vi "worker2.vi"(10 "user.xls path":path, 11 "Python version":string) -> (0 "error out":errorcluster, 8 "error In":errorcluster)   [LabVIEW 2020]
uses:
  status/stop software.vi
  status/skip_status.vi
  status/pause2.vi
  status/emergency stop.vi
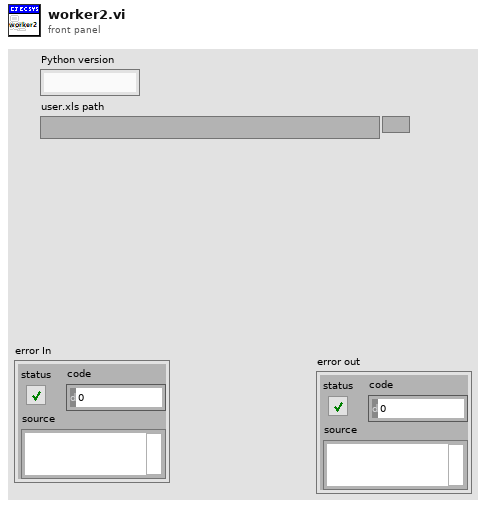
[diagram p1: front panel]
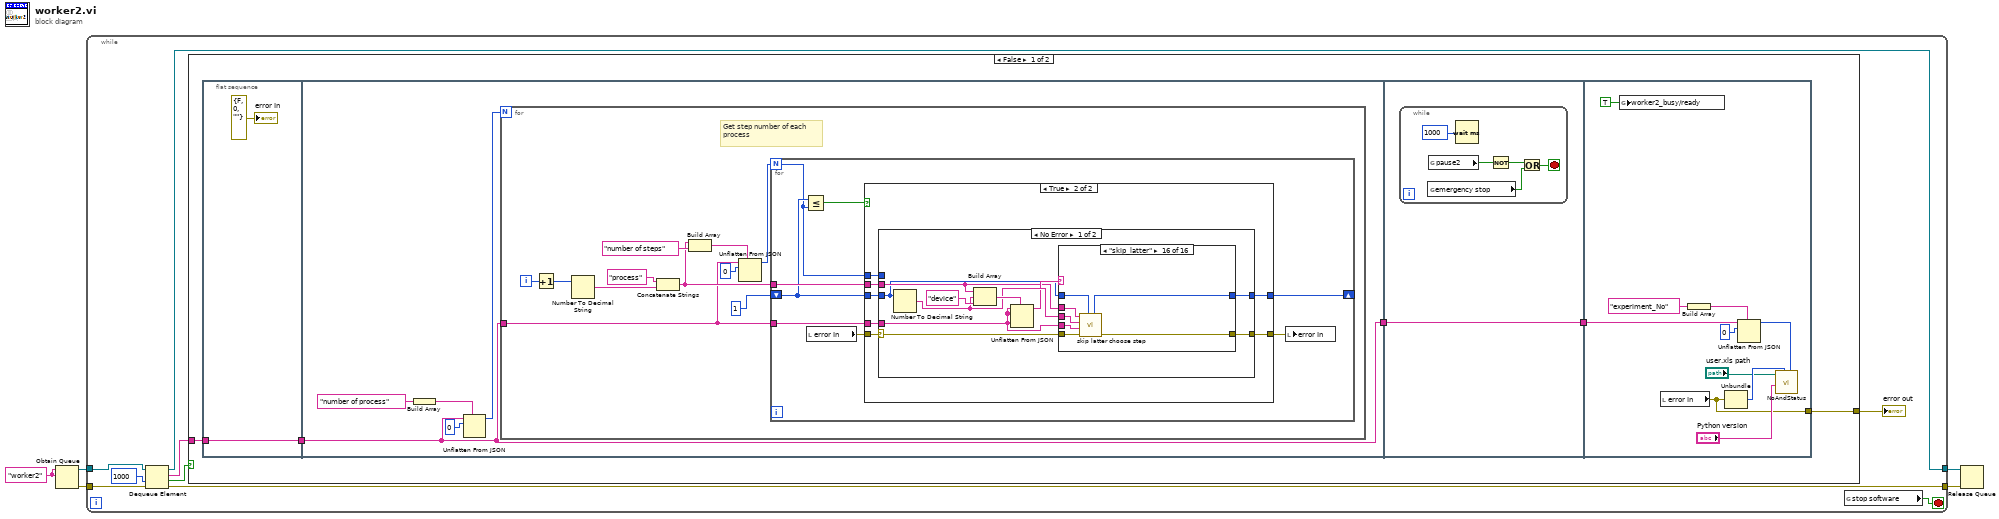
[diagram p0: block diagram]
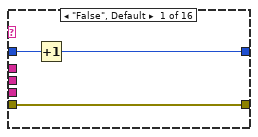
[diagram p3: hidden frame]
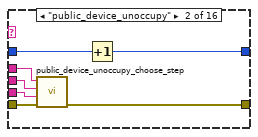
[diagram p4: hidden frame]
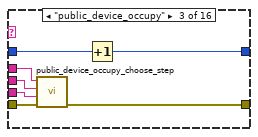
[diagram p5: hidden frame]
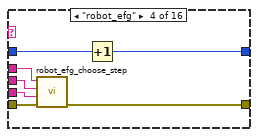
[diagram p6: hidden frame]
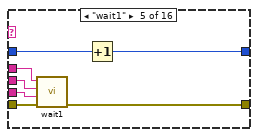
[diagram p7: hidden frame]
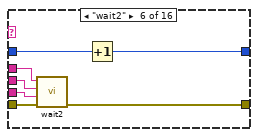
[diagram p8: hidden frame]
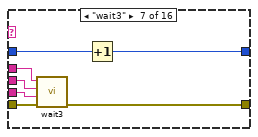
[diagram p9: hidden frame]
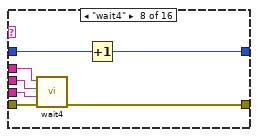
[diagram p10: hidden frame]
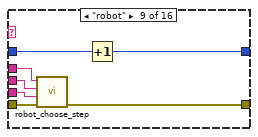
[diagram p11: hidden frame]
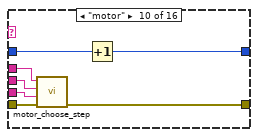
[diagram p12: hidden frame]
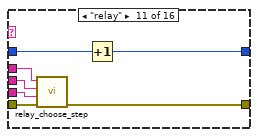
[diagram p13: hidden frame]
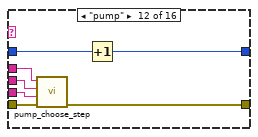
[diagram p14: hidden frame]
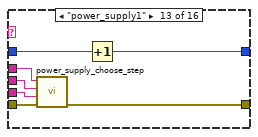
[diagram p15: hidden frame]
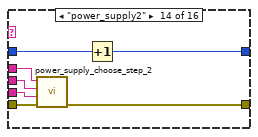
[diagram p16: hidden frame]
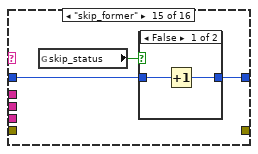
[diagram p17: hidden frame]
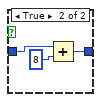
[diagram p18: hidden frame]
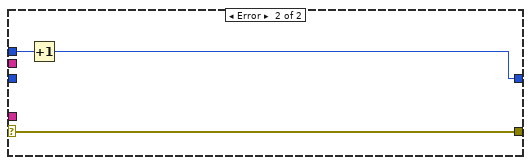
[diagram p19: hidden frame]
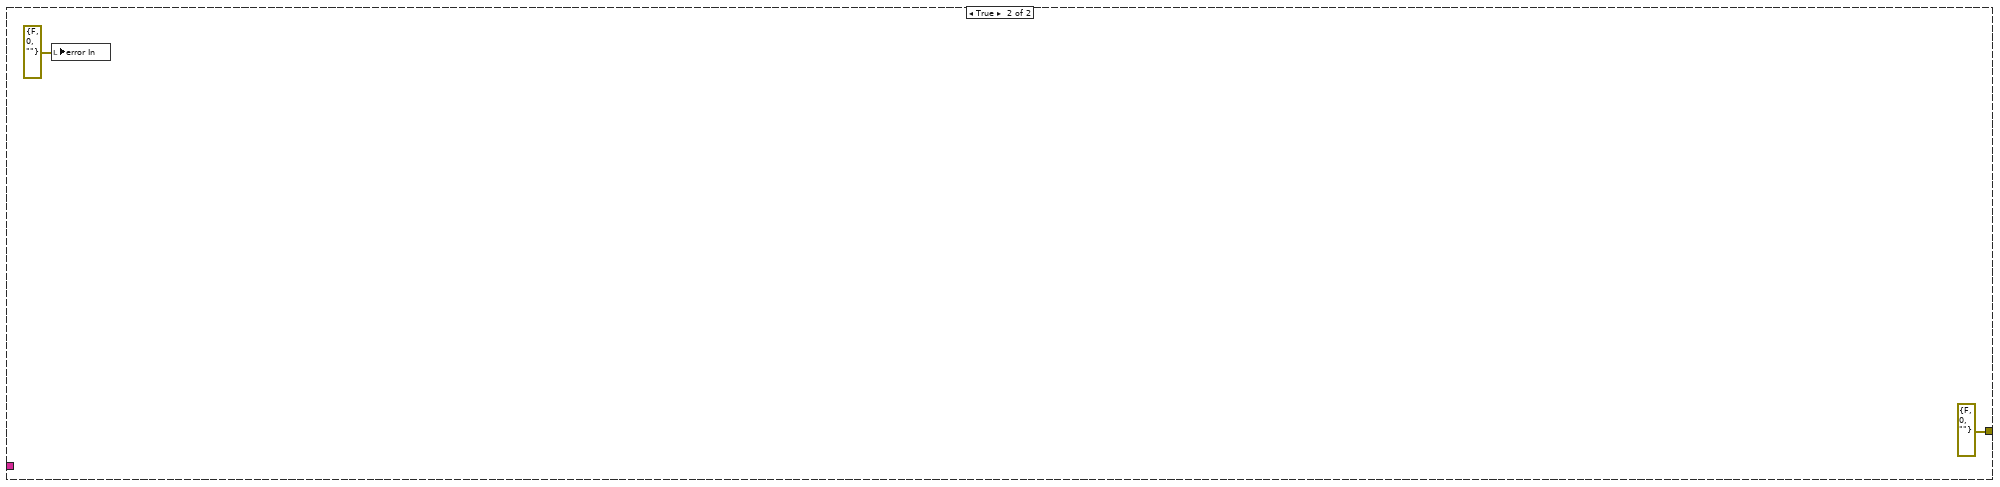
[diagram p20: hidden frame]
diagram:
  w3 = "worker2" ("name (unnamed)")
  n1 = Obtain Queue(name (unnamed)=w3, element data type=w3) -> (queue out=w2:refnum<queue>, error out=w1:errorcluster)  [unwired: 3 in, 1 out]
  n2 = while {
    tunnel: [w11] -> w5
    tunnel: [w10] -> w4
    tunnel: w2 -> [w7]
    tunnel: w1 -> [w6]
    stop <- w9 stop-if-true
    n3 = Dequeue Element(queue=w7, timeout in ms (-1)=1000, error in (no error)=w6) -> (queue out=w11:refnum<queue>, element=w12:string, timed out?=w14:bool, error out=w10:errorcluster)
    n4 = case shown="False" w14 {
      tunnel: w12 -> [w18 _]
      tunnel: [w15 errorcluster {"status"=FALSE, "code"=0, "source"=""} ("error In")] -> w8
      frame False {
        n5 = flat-sequence {
          tunnel: [w21] -> w19
          tunnel: w18 -> [w21]
          tunnel: w19 -> [w22]
          tunnel: [w22] -> w16
          tunnel: [w177] -> w17
          tunnel: w16 -> [w177]
          tunnel: w17 -> [w185]
          tunnel: [w183] -> w15
          frame #0 {
            "error In" <- errorcluster {"status"=FALSE, "code"=0, "source"=""} ("error In")
          }
          frame #1 {
            n6 = Build Array("number of process") -> (w24:string[])
            n7 = Unflatten From JSON(path=w24, JSON string=w22, type and defaults=0) -> (value=w23:i32)  [unwired: 4 in, 1 out]
            n8 = for {
              N: w23 -> [_]
              tunnel: w22 -> [w28]
              i -> [w35]
              # "Get step number of each process"
              n9 = Increment(x=w35) -> (x+1=w30:i32)
              n10 = Number To Decimal String(number=w30) -> (decimal integer string=w33:string)  [unwired: 1 in]
              n11 = Concatenate Strings("process" ("string"), w33) -> (w29:string)
              n12 = Build Array(w29, "number of steps" ("element")) -> (w31:string[])
              n13 = Unflatten From JSON(path=w31, JSON string=w28, type and defaults=0) -> (value=w36:i32)  [unwired: 4 in, 1 out]
              n14 = for {
                N: w36 -> [w38]
                tunnel: w29 -> [w43]
                tunnel: w28 -> [w42]
                shift-right: [w40] -> _
                shift-left: 1 ("Numeric") -> [w39]
                n15 = Less Or Equal?(x=w39, y=w38) -> (x <= y?=w41:bool)
                n16 = local read "error In"() -> (w45:errorcluster)
                n17 = case shown="True" w41 {
                  tunnel: [w47 w54] -> w44
                  tunnel: w45 -> [w47 w53]
                  tunnel: w42 -> [_ w52]
                  tunnel: w39 -> [w46 w51]
                  tunnel: [w46 w50] -> w40
                  tunnel: w38 -> [_ w49]
                  tunnel: w43 -> [_ w48]
                  frame False {
                  }
                  frame True {
                    n18 = case shown="No Error" w53 {
                      selector: w53 -> [w59 w176]
                      tunnel: [w63 w176] -> w54
                      tunnel: w48 -> [w58 _]
                      tunnel: w52 -> [w57 _]
                      tunnel: w51 -> [w55 _]
                      tunnel: [w56 w175] -> w50
                      tunnel: w49 -> [_ w174]
                      frame No Error {
                        n19 = Number To Decimal String(number=w55) -> (decimal integer string=w61:string)  [unwired: 1 in]
                        n20 = Build Array(w58, w61, "device" ("element")) -> (w62:string[])
                        n21 = Unflatten From JSON(path=w62, JSON string=w57, type and defaults=w57) -> (value=w60:string)  [unwired: 4 in, 1 out]
                        n22 = case shown="\"skip_latter\"" w60 {
                          tunnel: w57 -> [_ w71 w78 w88 w92 w99 w107 w114 w120 w127 w134 w144 w149 w155 _ w172]
                          tunnel: [w67 w74 w81 w87 w95 w102 w106 w113 w123 w130 w137 w143 w151 w158 _ w168] -> w63
                          tunnel: w61 -> [_ w72 w79 w85 w93 w100 w108 w115 w121 w128 w135 w141 w148 w156 _ w171]
                          tunnel: w58 -> [_ w73 w80 w86 w94 w101 w109 w116 w122 w129 w136 w142 w150 w157 _ w173]
                          tunnel: w59 -> [w67 w70 w77 w84 w91 w98 w105 w112 w119 w126 w133 w140 w147 w154 _ w167]
                          tunnel: [w66 w69 w76 w82 w90 w97 w104 w111 w118 w125 w132 w139 w146 w153 w159 w169] -> w56
                          tunnel: w55 -> [w65 w68 w75 w83 w89 w96 w103 w110 w117 w124 w131 w138 w145 w152 w160 w170]
                          frame "False", Default {
                            n23 = Increment(x=w65) -> (x+1=w66:i32)
                          }
                          frame "public_device_unoccupy" {
                            n24 = call "public_device_unoccupy_choose_step.vi"("error In"=w70, "JSON string"=w71, "Step order"=w72, "process_ID"=w73) -> ("error IO"=w74:errorcluster)  [unwired: 7 in]
                            n25 = Increment(x=w68) -> (x+1=w69:i32)
                          }
                          frame "public_device_occupy" {
                            n26 = call "public_device_occupy_choose_step.vi"("error In"=w77, "JSON string"=w78, "Step order"=w79, "process_ID"=w80) -> ("error IO"=w81:errorcluster)  [unwired: 7 in]
                            n27 = Increment(x=w75) -> (x+1=w76:i32)
                          }
                          frame "robot_efg" {
                            n28 = call "robot_efg_choose_step.vi"("error In"=w84, "JSON string"=w88, "Step order"=w85, "process_ID"=w86) -> ("error IO"=w87:errorcluster)  [unwired: 7 in]
                            n29 = Increment(x=w83) -> (x+1=w82:i32)
                          }
                          frame "wait1" {
                            n30 = call "wait1.vi"("error In"=w91, "JSON string"=w92, "Step order"=w93, "process_ID"=w94) -> ("error IO"=w95:errorcluster)  [unwired: 7 in]
                            n31 = Increment(x=w89) -> (x+1=w90:i32)
                          }
                          frame "wait2" {
                            n32 = call "wait2.vi"("error In"=w98, "JSON string"=w99, "Step order"=w100, "process_ID"=w101) -> ("error IO"=w102:errorcluster)  [unwired: 7 in]
                            n33 = Increment(x=w96) -> (x+1=w97:i32)
                          }
                          frame "wait3" {
                            n34 = call "wait3.vi"("error In"=w105, "JSON string"=w107, "Step order"=w108, "process_ID"=w109) -> ("error IO"=w106:errorcluster)  [unwired: 7 in]
                            n35 = Increment(x=w103) -> (x+1=w104:i32)
                          }
                          frame "wait4" {
                            n36 = call "wait4.vi"("error In"=w112, "JSON string"=w114, "Step order"=w115, "process_ID"=w116) -> ("error IO"=w113:errorcluster)  [unwired: 7 in]
                            n37 = Increment(x=w110) -> (x+1=w111:i32)
                          }
                          frame "robot" {
                            n38 = call "robot_choose_step.vi"("error In"=w119, "JSON string"=w120, "Step order"=w121, "process_ID"=w122) -> ("error IO"=w123:errorcluster)  [unwired: 7 in]
                            n39 = Increment(x=w117) -> (x+1=w118:i32)
                          }
                          frame "motor" {
                            n40 = call "motor_choose_step.vi"("error In"=w126, "JSON string"=w127, "Step order"=w128, "process_ID"=w129) -> ("error IO"=w130:errorcluster)  [unwired: 7 in]
                            n41 = Increment(x=w124) -> (x+1=w125:i32)
                          }
                          frame "relay" {
                            n42 = call "relay_choose_step.vi"("error In"=w133, "JSON string"=w134, "Step order"=w135, "process_ID"=w136) -> ("error IO"=w137:errorcluster)  [unwired: 7 in]
                            n43 = Increment(x=w131) -> (x+1=w132:i32)
                          }
                          frame "pump" {
                            n44 = call "pump_choose_step.vi"("error In"=w140, "JSON string"=w144, "Step order"=w141, "process_ID"=w142) -> ("error IO"=w143:errorcluster)  [unwired: 7 in]
                            n45 = Increment(x=w138) -> (x+1=w139:i32)
                          }
                          frame "power_supply1" {
                            n46 = call "power_supply_choose_step.vi"("error In"=w147, "JSON string"=w149, "Step order"=w148, "process_ID"=w150) -> ("error IO"=w151:errorcluster)  [unwired: 7 in]
                            n47 = Increment(x=w145) -> (x+1=w146:i32)
                          }
                          frame "power_supply2" {
                            n48 = call "power_supply_choose_step_2.vi"("error In"=w154, "JSON string"=w155, "Step order"=w156, "process_ID"=w157) -> ("error IO"=w158:errorcluster)  [unwired: 7 in]
                            n49 = Increment(x=w152) -> (x+1=w153:i32)
                          }
                          frame "skip_former" {
                            n50 = global read "skip_status.vi" "skip_status"() -> (w161:bool)
                            n51 = case shown="False" w161 {
                              tunnel: w160 -> [w162 w166]
                              tunnel: [w163 w164] -> w159
                              frame False {
                                n52 = Increment(x=w162) -> (x+1=w163:i32)
                              }
                              frame True {
                                n53 = Add(x=w166, y=8) -> (x+y=w164:i32)
                              }
                            }
                          }
                          frame "skip_latter" {
                            n54 = call "skip latter choose step.vi"("step number"=w170, "error In"=w167, "JSON string"=w172, "Step order"=w171, "process_ID"=w173) -> ("error IO"=w168:errorcluster, "step number after"=w169:i32)  [unwired: 5 in]
                          }
                        }
                      }
                      frame Error {
                        n55 = Increment(x=w174) -> (x+1=w175:i32)
                      }
                    }
                  }
                }
                n56 = local write "error In"(w44) -> ()
              }
            }
          }
          frame #2 {
            n57 = while {
              stop <- w179 stop-if-true
              n58 = global read "emergency stop.vi" "emergency stop"() -> (w181:bool)
              n59 = global read "pause2.vi" "pause2"() -> (w182:bool)
              n60 = Wait (ms)(milliseconds to wait=u32 1000) -> ()  [unwired: 1 out]
              n61 = Not(x=w182) -> (.not. x?=w180:bool)
              n62 = Or(x=w180, y=w181) -> (x .or. y?=w179:bool)
            }
          }
          frame #3 {
            n63 = global write "status of worker2.vi" "worker2_busy/ready"(TRUE ("worker2_busy/ready")) -> ()
            n64 = local read "error In"() -> (w183:errorcluster)
            n65 = Build Array("experiment_No") -> (w186:string[])
            n66 = Unbundle(w183) -> ("code"=w190:i32)  [unwired: 2 out]
            n67 = Unflatten From JSON(path=w186, JSON string=w185, type and defaults=0) -> (value=w184:i32)  [unwired: 4 in, 1 out]
            n68 = call "NoAndStatus.vi"("experiment_no"=w184, "vial_no"=w190, "Python version"="Python version", "user.xls path"="user.xls path") -> ()  [unwired: 7 in, 1 out]
          }
        }
      }
      frame True {
        n69 = local write "error In"(errorcluster {"status"=FALSE, "code"=0, "source"=""} ("error In")) -> ()
      }
    }
    "error out" <- w8
    n70 = global read "stop software.vi" "stop software"() -> (w9:bool)
  }
  n71 = Release Queue(queue=w5, error in (no error)=w4) -> ()  [unwired: 1 in, 3 out]
